vi "Dialog Selector SIC.vi"(11 "error in (no error)":errorcluster) -> (8 "Dialog Selector Q":refnum<queue>, 15 "error out":errorcluster)   [LabVIEW 2011]
uses:
  Dialog selection cluster.ctl
  Dialog box ID.ctl
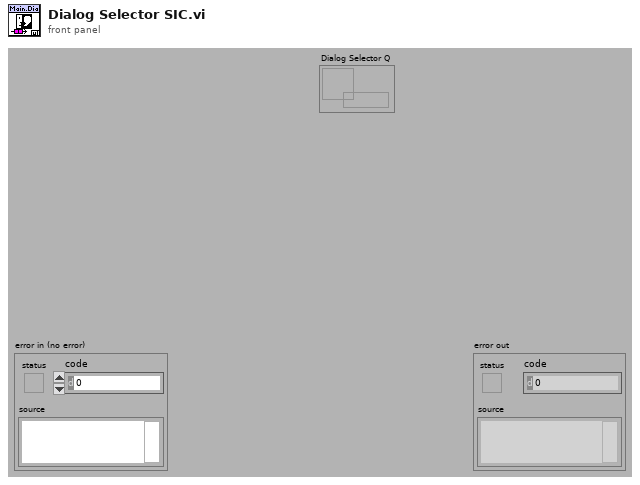
[diagram p1: front panel]
types:
  T1 = typedef "Dialog selection cluster.ctl" = cluster{"ID":T2, "Details":variant}
  T2 = typedef "Dialog box ID.ctl" = enum16{"About dialog Box", "Options dialog box", "User dialog Box", "Custom dialog...", "Variables Common Analog", "Annotation", "Welcome screen", "Variables Tool Analog", "High G graph display", "Sequence setup", "Unused"}
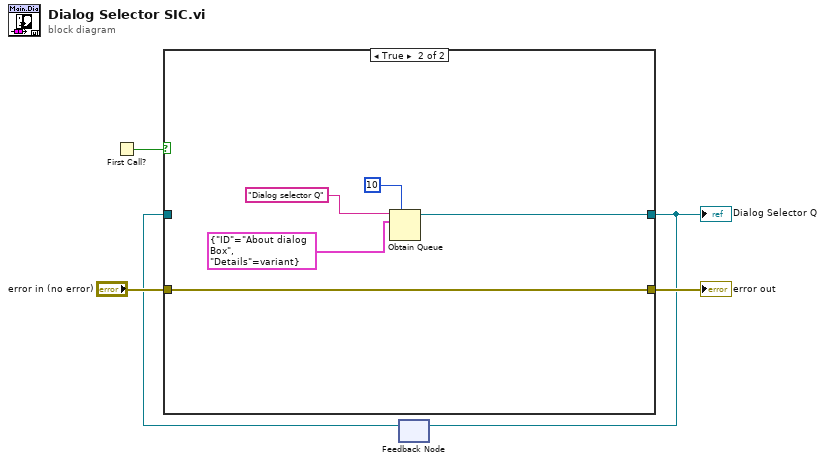
[diagram p0: block diagram]
diagram:
  n1 = First Call?() -> (First Call?: T/F=w3:bool)
  n2 = feedback #1() -> (w1:refnum<queue>)  [unwired: 1 in]
  n3 = case shown="True" w3 {
    tunnel: [w7 w12] -> w5
    tunnel: "error in (no error)" -> [w7 w12]
    tunnel: [w6 w11] -> w2
    tunnel: w1 -> [w6 _]
    frame False {
    }
    frame True {
      n4 = Obtain Queue(max queue size (-1, unlimited)=10, name (unnamed)="Dialog selector Q", element data type=T1 {"ID"=enum."About dialog Box", "Details"=variant} ("Cluster")) -> (queue out=w11:refnum<queue>)  [unwired: 2 in, 2 out]
    }
  }
  "error out" <- w5
  "Dialog Selector Q" <- w2
  n5 = feedback-in #1(w2) -> ()
